vi "readTiff.vi"(10 "file (use dialog)":path=path "C:/Users/Administrator/Desktop/test.tiff") -> (1 "Vss":sgl, 2 "HSS":u32, 3 "imageHeight":i32, 5 "imageWidth":i32)   [LabVIEW 2016]
uses:
  subVIs/variables/imageSettings.vi
panel:
  out "size (in bytes)":i64
  out "Intensity Graph 2":i32[][](graph)
  out "Intensity Graph":i32[][](graph)
  out "String":string
  out "offsetTo5277":u32
  out "imageDataType":u16
  out "stripCount":u32
  out "stripOffset":u32
  out "pixelDim":i32
  out "TAG Format":T1={"ID"=0, "Data Type"=enum."U8", "Data Count"=0, "Data Value"=0}
  out "arrayLength":i32
  out "byteToFirstIfd":u32
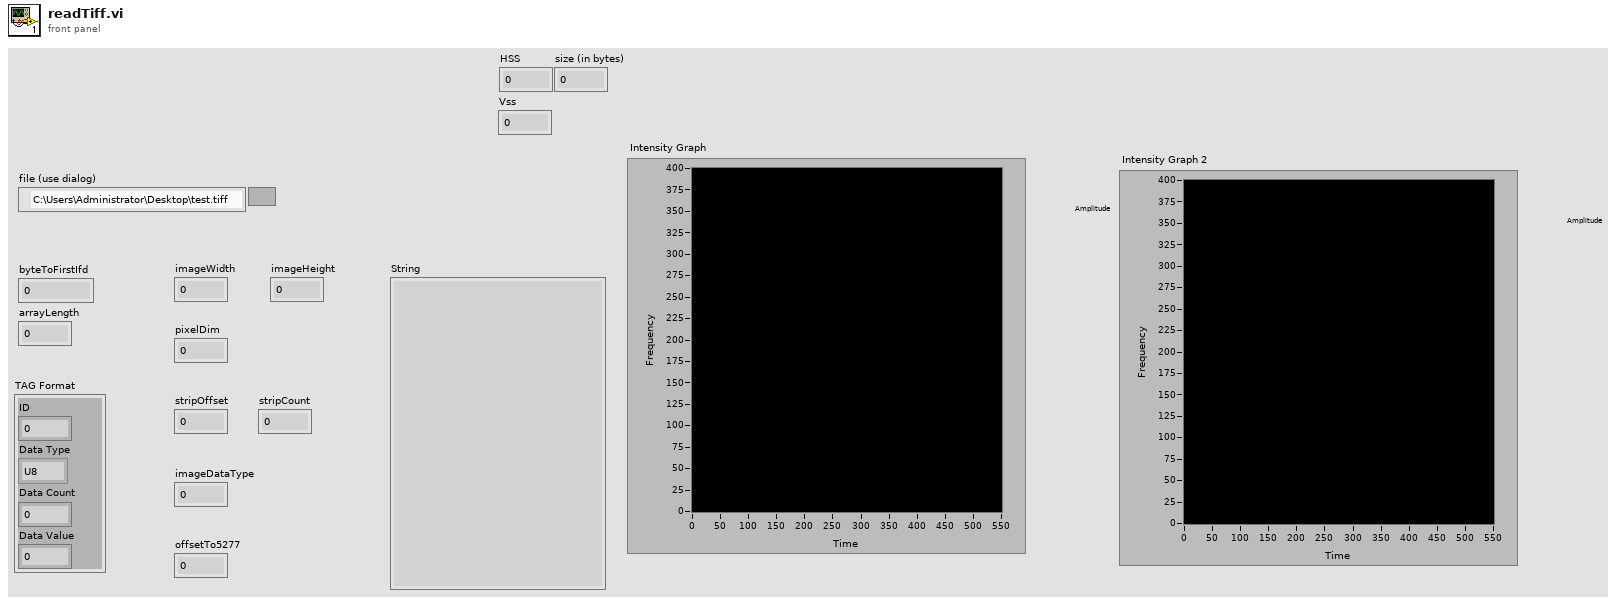
[diagram p1: front panel]
types:
  T1 = cluster{"ID":u16, "Data Type":enum16{"Undefined(DO NOT USE)", "U8", "ASCII", "U16", "U32", "RATIONAL", "I8", "Undefined 8 bit", "I16", "I32", "SRATIONAL", "SGL", "DBL"}, "Data Count":u32, "Data Value":u32}
  T2 = enum16{"big-endian, network order", "native, host order", "little-endian"}
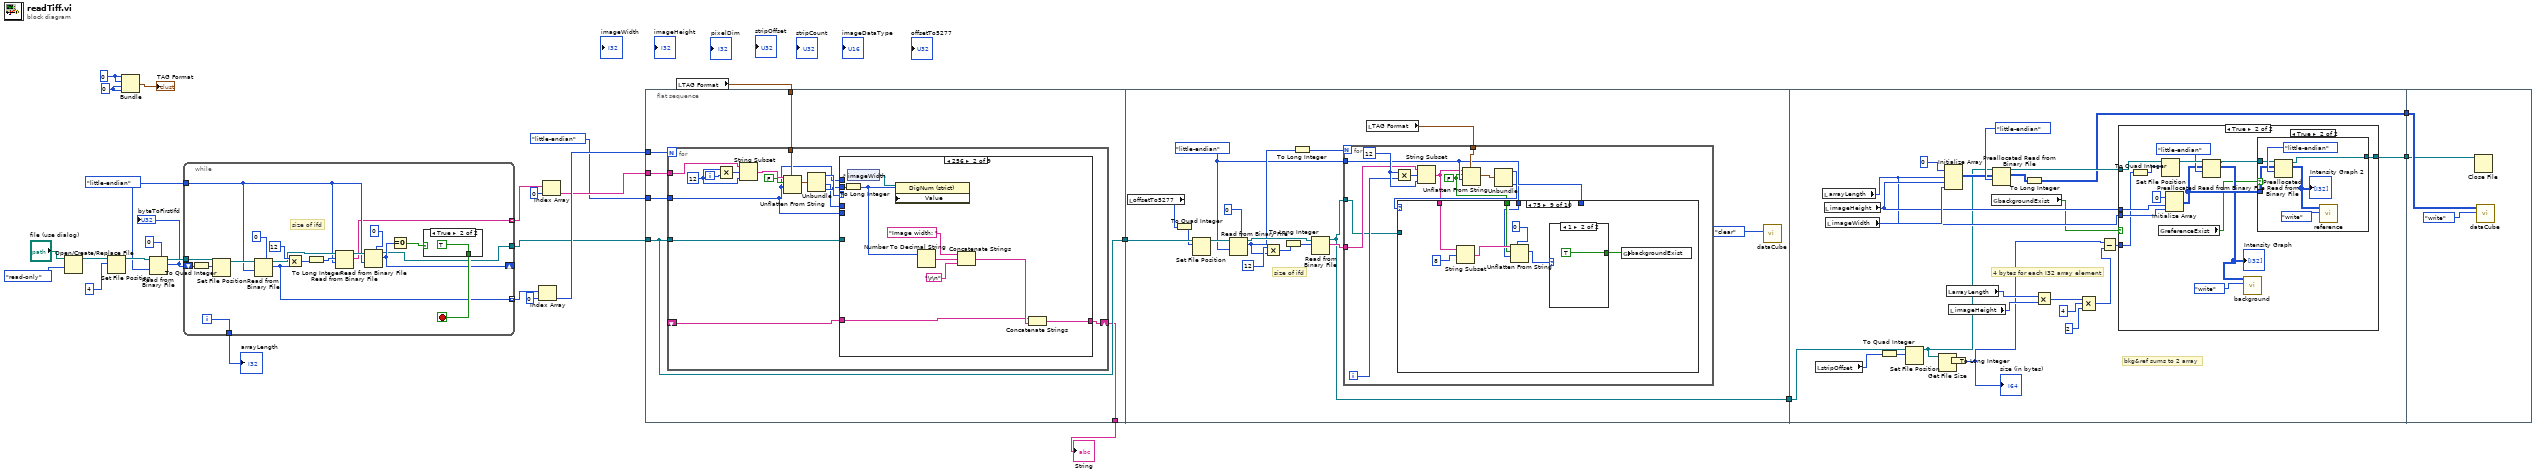
[diagram p0: block diagram]
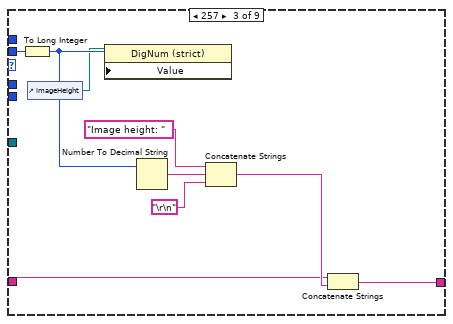
[diagram p3: hidden frame]
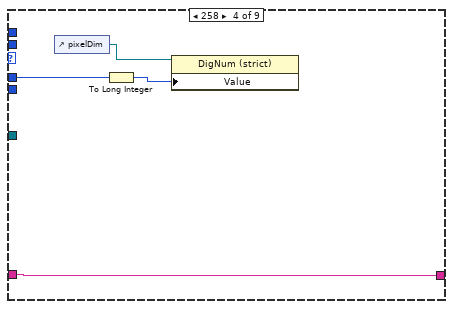
[diagram p4: hidden frame]
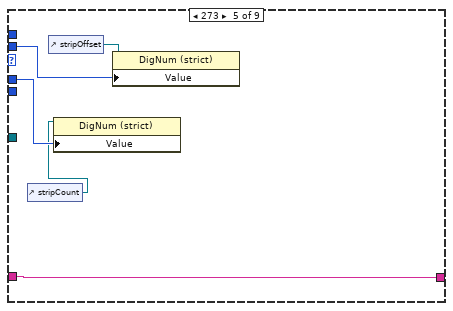
[diagram p5: hidden frame]
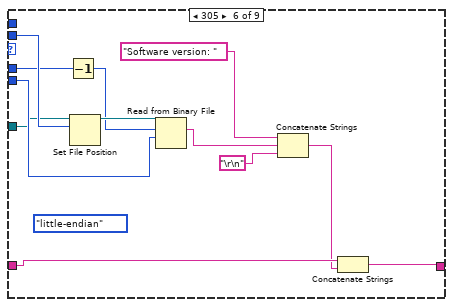
[diagram p6: hidden frame]
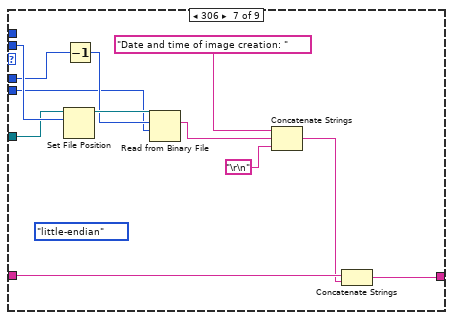
[diagram p7: hidden frame]
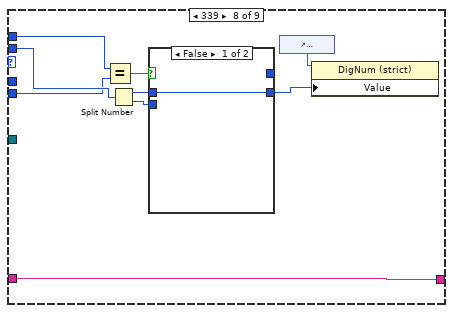
[diagram p8: hidden frame]
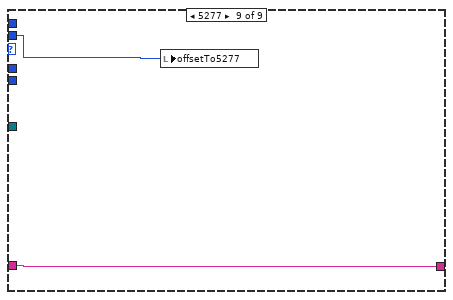
[diagram p10: hidden frame]
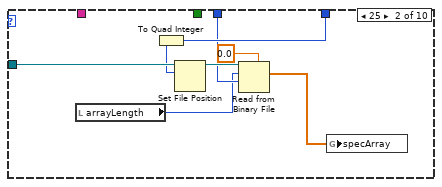
[diagram p12: hidden frame]
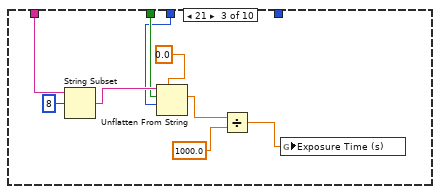
[diagram p13: hidden frame]
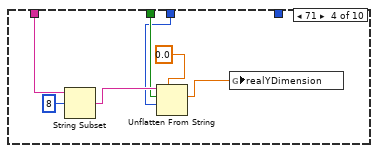
[diagram p14: hidden frame]
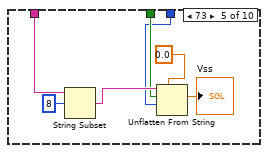
[diagram p15: hidden frame]
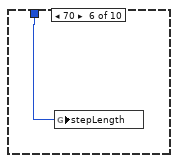
[diagram p16: hidden frame]
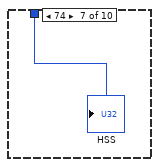
[diagram p17: hidden frame]
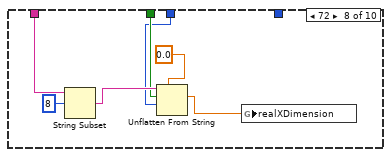
[diagram p18: hidden frame]
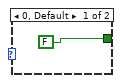
[diagram p19: hidden frame]
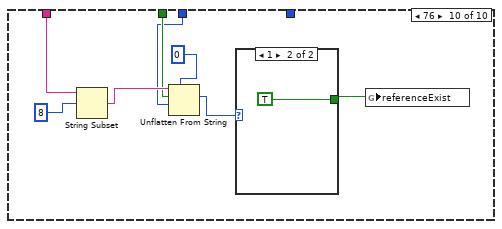
[diagram p20: hidden frame]
diagram:
  w17 = u32 0
  w18 = u16 0
  w20 = T2."little-endian" ("byte order (0:big-endian, network order)")
  n1 = Open/Create/Replace File(file path (use dialog)="file (use dialog)", access (0:read/write)=enum16{"read/write", "read-only", "write-only"}."read-only") -> (refnum out=w25:refnum<file>)  [unwired: 4 in, 2 out]
  n2 = Set File Position(offset (in bytes) (0)=i64 4, refnum=w25) -> (refnum out=w27:refnum<file>)  [unwired: 2 in, 1 out]
  n3 = Bundle(w18, w18, w17, w17) -> (→"TAG Format":cluster{u16, u16, u32, u32})  [unwired: 1 in]
  n4 = Read from Binary File(5:u32 0, 9:w20, 11:w27) -> (2:w19:u32, 3:w21:refnum<file>)  [unwired: 3 in, 2 out]
  "byteToFirstIfd" <- w19
  n5 = while {
    tunnel: w20 -> [w38]
    shift-right: [w31] -> _
    shift-left: w19 -> [w35]
    tunnel: [w33] -> w15 mode=indexing
    tunnel: w21 -> [w46]
    tunnel: [w30] -> w5
    tunnel: [w29] -> w13 mode=indexing
    tunnel: [w28] -> w11
    i -> [w28]
    stop <- w32 stop-if-true
    # "size of ifd"
    n6 = To Quad Integer(1:w35) -> (0:w34:i64)
    n7 = Set File Position(offset (in bytes) (0)=w34, refnum=w46) -> (refnum out=w45:refnum<file>)  [unwired: 2 in, 1 out]
    n8 = Read from Binary File(5:u16 0, 9:w38, 11:w45) -> (2:w29:u16, 3:w40:refnum<file>)  [unwired: 3 in, 2 out]
    n9 = Multiply(x=u16 12, y=w29) -> (x*y=w42:u16)
    n10 = To Long Integer(number=w42) -> (32bit integer=w41:i32)
    n11 = Read from Binary File(9:w38, 10:w41, 11:w40) -> (2:w33:string, 3:w39:refnum<file>)  [unwired: 3 in, 2 out]
    n12 = Read from Binary File(5:u32 0, 9:w38, 11:w39) -> (2:w31:u32, 3:w30:refnum<file>)  [unwired: 3 in, 2 out]
    n13 = Equal To 0?(x=w31) -> (x = 0?=w36:bool)
    n14 = case shown="True" w36 {
      tunnel: [FALSE TRUE] -> w32
      frame False {
      }
      frame True {
      }
    }
  }
  "arrayLength" <- w11
  n15 = Index Array(array=w13, index=0) -> (element=w8:u16)
  n16 = Index Array(array=w15, index=0) -> (element=w7:string)
  n17 = flat-sequence {
    tunnel: w5 -> [w50]
    tunnel: [w50] -> w10
    tunnel: w9 -> [w54]
    tunnel: w8 -> [w53]
    tunnel: w7 -> [w52]
    tunnel: T2."little-endian" ("byte order") -> [w51]
    tunnel: [w49] -> w4
    tunnel: w10 -> [w151]
    tunnel: [w137] -> w3
    tunnel: w3 -> [w246]
    tunnel: [w226] -> w2
    tunnel: [w225] -> w1
    tunnel: w2 -> [w272]
    tunnel: w1 -> [w270]
    frame #0 {
      n18 = for {
        N: w53 -> [_]
        tunnel: w52 -> [w68]
        tunnel: w54 -> [w62]
        tunnel: w51 -> [w56]
        shift-right: [w58] -> w49
        shift-left: _ -> [w59]
        tunnel: w50 -> [w55]
        i -> [w69]
        w67 = 12 ("x")
        n19 = Multiply(x=w67, y=w69) -> (x*y=w66:i32)
        n20 = String Subset(string=w68, offset (0)=w66, length (rest)=w67) -> (substring=w57:string)
        n21 = Unflatten From String(type=w62, binary string=w57, data includes array or string size? (T)=FALSE, byte order (0:big-endian, network order)=w56) -> (value=w61:T1)  [unwired: 1 in, 2 out]
        n22 = Unbundle(w61) -> ("ID"=w65:u16, "Data Count"=w63:u32, "Data Value"=w64:u32)  [unwired: 1 out]
        n23 = case shown="256" w65 {
          tunnel: w64 -> [_ w79 w88 _ w96 w105 w119 w130 w134]
          tunnel: w63 -> [_ _ _ w92 w97 w104 w118 _ _]
          tunnel: w56 -> [_ _ _ _ _ _ _ w129 _]
          tunnel: w56 -> [_ _ _ _ _ w99 w111 w128 _]
          tunnel: w59 -> [w70 w73 w83 w90 w95 w102 w116 w123 w135]
          tunnel: [w70 w72 w82 w90 w95 w103 w117 w123 w135] -> w58
          tunnel: w55 -> [_ _ _ _ _ w98 w110 _ _]
          frame Default {
          }
          frame 256 {
            n24 = To Long Integer(number=w79) -> (32bit integer=w77:i32)
            n25 = control-ref of="imageWidth"() -> (w71:refnum<vi>)
            n26 = property on="Property Node" class="DigNum (strict)"(reference=w71, "Value"=w77) -> ()  [unwired: 1 in, 2 out]
            n27 = Number To Decimal String(number=w77) -> (decimal integer string=w76:string)  [unwired: 1 in]
            n28 = Concatenate Strings("Image width: ", w76, "\r\n") -> (w74:string)
            n29 = Concatenate Strings(w73, w74) -> (w72:string)
          }
          frame 257 {
            n30 = To Long Integer(number=w88) -> (32bit integer=w81:i32)
            n31 = control-ref of="imageHeight"() -> (w80:refnum<vi>)
            n32 = property on="Property Node" class="DigNum (strict)"(reference=w80, "Value"=w81) -> ()  [unwired: 1 in, 2 out]
            n33 = Number To Decimal String(number=w81) -> (decimal integer string=w86:string)  [unwired: 1 in]
            n34 = Concatenate Strings("Image height: ", w86, "\r\n") -> (w84:string)
            n35 = Concatenate Strings(w83, w84) -> (w82:string)
          }
          frame 258 {
            n36 = control-ref of="pixelDim"() -> (w89:refnum<vi>)
            n37 = To Long Integer(number=w92) -> (32bit integer=w91:i32)
            n38 = property on="Property Node" class="DigNum (strict)"(reference=w89, "Value"=w91) -> ()  [unwired: 1 in, 2 out]
          }
          frame 273 {
            n39 = control-ref of="stripCount"() -> (w93:refnum<vi>)
            n40 = control-ref of="stripOffset"() -> (w94:refnum<vi>)
            n41 = property on="Property Node" class="DigNum (strict)"(reference=w93, "Value"=w97) -> ()  [unwired: 1 in, 2 out]
            n42 = property on="Property Node" class="DigNum (strict)"(reference=w94, "Value"=w96) -> ()  [unwired: 1 in, 2 out]
          }
          frame 305 {
            (unwired) T2."little-endian" ("byte order (0:big-endian, network order)")
            n43 = Decrement(x=w104) -> (x-1=w108:u32)
            n44 = Set File Position(offset (in bytes) (0)=w105, refnum=w98) -> (refnum out=w109:refnum<file>)  [unwired: 2 in, 1 out]
            n45 = Read from Binary File(9:w99, 10:w108, 11:w109) -> (2:w106:string)  [unwired: 3 in, 3 out]
            n46 = Concatenate Strings("Software version: ", w106, "\r\n") -> (w101:string)
            n47 = Concatenate Strings(w102, w101) -> (w103:string)
          }
          frame 306 {
            (unwired) T2."little-endian" ("byte order (0:big-endian, network order)")
            n48 = Set File Position(offset (in bytes) (0)=w119, refnum=w110) -> (refnum out=w121:refnum<file>)  [unwired: 2 in, 1 out]
            n49 = Decrement(x=w118) -> (x-1=w120:u32)
            n50 = Read from Binary File(9:w111, 10:w120, 11:w121) -> (2:w114:string)  [unwired: 3 in, 3 out]
            n51 = Concatenate Strings("Date and time of image creation: ", w114, "\r\n") -> (w113:string)
            n52 = Concatenate Strings(w116, w113) -> (w117:string)
          }
          frame 339 {
            n53 = Equal?(x=w129, y=w128) -> (x = y?=w127:bool)
            n54 = Split Number(x=w130) -> (hi(x)=w124:u16, lo(x)=w125:u16)
            n55 = case shown="False" w127 {
              tunnel: [w131 w133] -> w126
              tunnel: w125 -> [_ w133]
              tunnel: w124 -> [w131 w132]
              tunnel: [_ w132] -> _
              frame False {
              }
              frame True {
              }
            }
            n56 = control-ref of="imageDataType"() -> (w122:refnum<vi>)
            n57 = property on="Property Node" class="DigNum (strict)"(reference=w122, "Value"=w126) -> ()  [unwired: 1 in, 2 out]
          }
          frame 5277 {
            n58 = local write "offsetTo5277"(w134) -> ()
          }
        }
      }
    }
    frame #1 {
      w140 = T2."little-endian" ("byte order (0:big-endian, network order)")
      # "size of ifd"
      n59 = local read "offsetTo5277"() -> (w138:u32)
      n60 = To Quad Integer(1:w138) -> (0:w139:i64)
      n61 = Set File Position(offset (in bytes) (0)=w139, refnum=w151) -> (refnum out=w150:refnum<file>)  [unwired: 2 in, 1 out]
      n62 = Read from Binary File(5:u16 0, 9:w140, 11:w150) -> (2:w143:u16, 3:w145:refnum<file>)  [unwired: 3 in, 2 out]
      n63 = Multiply(x=u16 12, y=w143) -> (x*y=w147:u16)
      n64 = To Long Integer(number=w147) -> (32bit integer=w146:i32)
      n65 = To Long Integer(number=w143) -> (32bit integer=w142:i32)
      n66 = Read from Binary File(10:w146, 11:w145) -> (2:w144:string, 3:w137:refnum<file>)  [unwired: 4 in, 2 out]
      n67 = local read "TAG Format"() -> (w141:T1)
      n68 = for {
        N: w142 -> [_]
        tunnel: w144 -> [w160]
        tunnel: w137 -> [w156]
        tunnel: w141 -> [w159]
        tunnel: w140 -> [w154]
        i -> [w158]
        w152 = FALSE ("data includes array or string size? (T)")
        w163 = 12 ("x")
        n69 = Multiply(x=w163, y=w158) -> (x*y=w162:i32)
        n70 = String Subset(string=w160, offset (0)=w162, length (rest)=w163) -> (substring=w153:string)
        n71 = Unflatten From String(type=w159, binary string=w153, data includes array or string size? (T)=w152, byte order (0:big-endian, network order)=w154) -> (value=w161:T1)  [unwired: 1 in, 2 out]
        n72 = Unbundle(w161) -> ("ID"=w157:u16, "Data Value"=w155:u32)  [unwired: 2 out]
        n73 = case shown="75" w157 {
          tunnel: w156 -> [_ w171 _ _ _ _ _ _ _ _]
          tunnel: w155 -> [_ w170 _ _ _ w195 w196 _ _ _]
          tunnel: w154 -> [_ w168 w176 w183 w190 _ _ w199 w207 w217]
          tunnel: w153 -> [_ _ w180 w187 w194 _ _ w203 w211 w221]
          tunnel: w152 -> [_ _ w177 w184 w191 _ _ w200 w208 w218]
          frame 0, Default {
          }
          frame 25 {
            n74 = local read "arrayLength"() -> (w166:i32)
            n75 = To Quad Integer(1:w170) -> (0:w165:i64)
            n76 = Set File Position(offset (in bytes) (0)=w165, refnum=w171) -> (refnum out=w169:refnum<file>)  [unwired: 2 in, 1 out]
            n77 = Read from Binary File(5:sgl 0.0, 9:w168, 10:w166, 11:w169) -> (2:w164:sgl[])  [unwired: 2 in, 3 out]
            n78 = global write "imageSettings.vi" "specArray"(w164) -> ()
          }
          frame 21 {
            n79 = String Subset(string=w180, offset (0)=8) -> (substring=w178:string)  [unwired: 1 in]
            n80 = Unflatten From String(type=sgl 0.0, binary string=w178, data includes array or string size? (T)=w177, byte order (0:big-endian, network order)=w176) -> (value=w174:sgl)  [unwired: 1 in, 2 out]
            n81 = Divide(x=w174, y=sgl 1000.0) -> (x/y=w173:sgl)
            n82 = global write "imageSettings.vi" "Exposure Time (s)"(w173) -> ()
          }
          frame 71 {
            n83 = String Subset(string=w187, offset (0)=8) -> (substring=w185:string)  [unwired: 1 in]
            n84 = Unflatten From String(type=sgl 0.0, binary string=w185, data includes array or string size? (T)=w184, byte order (0:big-endian, network order)=w183) -> (value=w181:sgl)  [unwired: 1 in, 2 out]
            n85 = global write "imageSettings.vi" "realYDimension"(w181) -> ()
          }
          frame 73 {
            n86 = String Subset(string=w194, offset (0)=8) -> (substring=w192:string)  [unwired: 1 in]
            n87 = Unflatten From String(type=sgl 0.0, binary string=w192, data includes array or string size? (T)=w191, byte order (0:big-endian, network order)=w190) -> (value=→"Vss":sgl)  [unwired: 1 in, 2 out]
          }
          frame 70 {
            n88 = global write "imageSettings.vi" "stepLength"(w195) -> ()
          }
          frame 74 {
            "HSS" <- w196
          }
          frame 72 {
            n89 = String Subset(string=w203, offset (0)=8) -> (substring=w201:string)  [unwired: 1 in]
            n90 = Unflatten From String(type=sgl 0.0, binary string=w201, data includes array or string size? (T)=w200, byte order (0:big-endian, network order)=w199) -> (value=w197:sgl)  [unwired: 1 in, 2 out]
            n91 = global write "imageSettings.vi" "realXDimension"(w197) -> ()
          }
          frame 75 {
            n92 = String Subset(string=w211, offset (0)=8) -> (substring=w209:string)  [unwired: 1 in]
            n93 = Unflatten From String(type=u8 0, binary string=w209, data includes array or string size? (T)=w208, byte order (0:big-endian, network order)=w207) -> (value=w205:u8)  [unwired: 1 in, 2 out]
            n94 = case shown="1" w205 {
              tunnel: [FALSE TRUE] -> w204
              frame 0, Default {
              }
              frame 1 {
              }
            }
            n95 = global write "imageSettings.vi" "backgroundExist"(w204) -> ()
          }
          frame 76 {
            n96 = String Subset(string=w221, offset (0)=8) -> (substring=w219:string)  [unwired: 1 in]
            n97 = Unflatten From String(type=u8 0, binary string=w219, data includes array or string size? (T)=w218, byte order (0:big-endian, network order)=w217) -> (value=w215:u8)  [unwired: 1 in, 2 out]
            n98 = case shown="1" w215 {
              tunnel: [FALSE TRUE] -> w214
              frame 0, Default {
              }
              frame 1 {
              }
            }
            n99 = global write "imageSettings.vi" "referenceExist"(w214) -> ()
          }
        }
      }
      n100 = call "dataCube.vi"("Enum"=enum16{"clear", "read", "write"}."clear") -> ()  [unwired: 8 in, 3 out]
    }
    frame #2 {
      # "bkg&ref sums to 2 array"
      # "4 bytes for each I32 array element"
      n101 = local read "stripOffset"() -> (w245:u32)
      n102 = local read "arrayLength"() -> (w238:i32)
      n103 = local read "imageHeight"() -> (w239:i32)
      n104 = local read "imageWidth"() -> (w240:i32)
      n105 = To Quad Integer(1:w245) -> (0:w244:i64)
      n106 = Set File Position(offset (in bytes) (0)=w244, refnum=w246) -> (refnum out=w237:refnum<file>)  [unwired: 2 in, 1 out]
      n107 = Get File Size(file=w237) -> (size (in bytes)=w230:i64)  [unwired: 1 in, 2 out]
      n108 = Initialize Array(u16 0 ("element"), w238, w239, w240) -> (w242:u16[][][])
      n109 = local read "arrayLength"() -> (w235:i32)
      n110 = local read "imageHeight"() -> (w234:i32)
      n111 = To Long Integer(number=w230) -> (32bit integer=w228:i32)
      "size (in bytes)" <- w228
      n112 = global read "imageSettings.vi" "backgroundExist"() -> (w224:bool)
      n113 = Preallocated Read from Binary File(5:T2."little-endian" ("byte order (0:big-endian, network order)"), 6:w242, 7:w237) -> (2:w236:u16[][][], 3:w241:refnum<file>)  [unwired: 1 in, 2 out]
      n114 = To Long Integer(number=w236) -> (32bit integer=w226:i32[][][])
      n115 = Multiply(x=w235, y=w234) -> (x*y=w233:i32)
      n116 = Compound Arithmetic op=MULTIPLY(w233, 4 ("value"), 2 ("value")) -> (w229:i32)
      n117 = Subtract(x=w228, y=w229) -> (x-y=w227:i32)
      n118 = case shown="True" w224 {
        tunnel: w241 -> [w248 w262]
        tunnel: w239 -> [_ w261]
        tunnel: w238 -> [_ w260]
        tunnel: w227 -> [_ w254]
        tunnel: [w248 w250] -> w225
        frame False {
        }
        frame True {
          n119 = To Quad Integer(1:w254) -> (0:w253:i64)
          n120 = global read "imageSettings.vi" "referenceExist"() -> (w249:bool)
          n121 = Set File Position(offset (in bytes) (0)=w253, refnum=w262) -> (refnum out=w258:refnum<file>)  [unwired: 2 in, 1 out]
          n122 = Initialize Array(0 ("element"), w261, w260) -> (w255:i32[][])
          n123 = Preallocated Read from Binary File(5:T2."little-endian" ("byte order (0:big-endian, network order)"), 6:w255, 7:w258) -> (2:w252:i32[][], 3:w256:refnum<file>)  [unwired: 1 in, 2 out]
          "Intensity Graph" <- w252
          n124 = call "background.vi"("Enum"=enum16{"clear", "read", "write"}."write", "backgroundImageIn"=w252) -> ()  [unwired: 9 in, 1 out]
          n125 = case shown="True" w249 {
            tunnel: w256 -> [w263 w268]
            tunnel: w255 -> [_ w267]
            tunnel: [w263 w264] -> w250
            frame False {
            }
            frame True {
              n126 = Preallocated Read from Binary File(5:T2."little-endian" ("byte order (0:big-endian, network order)"), 6:w267, 7:w268) -> (2:w266:i32[][], 3:w264:refnum<file>)  [unwired: 1 in, 2 out]
              "Intensity Graph 2" <- w266
              n127 = call "reference.vi"("Enum"=enum16{"clear", "read", "write"}."write", "referenceImageIn"=w266) -> ()  [unwired: 9 in, 1 out]
            }
          }
        }
      }
    }
    frame #3 {
      n128 = Close File(refnum=w270) -> ()  [unwired: 1 in, 2 out]
      n129 = call "dataCube.vi"("Enum"=enum16{"clear", "read", "write"}."write", "imageCube"=w272) -> ()  [unwired: 7 in, 3 out]
    }
  }
  n130 = local read "TAG Format"() -> (w9:T1)
  "String" <- w4
